vi "MGCC_StaEst_idx2pha.vi"(1 "n":dbl, 2 "Index":dbl[](array[numeric])) -> (0 "byphase":dbl[][](array[numeric]))   [LabVIEW 2016]
uses:
  <vilib>/imath/engines/lvmath2/RunTimeEngine/BitwiseOperatorToken/NIMS_Bitwise_Operator_And.vi
  <instcachedir>/0/NIMS_Bitwise_Operator_And_D587B28D2F2E4A5ABF81AE0392B9AD1B.lvgen/NIMS_Bitwise_Operator_And_D587B28D2F2E4A5ABF81AE0392B9AD1B_001.vi
  <vilib>/imath/engines/lvmath2/RunTimeEngine/BuiltInFunctions/findnz/NIMS_[1o]_findnz(GRowV).vi
  <instcachedir>/0/NIMS_[1o]_findnz(GRowV)_1AF74843B4874134ADE908C0A4A72F3C.lvgen/NIMS_[1o]_findnz(GRowV)_1AF74843B4874134ADE908C0A4A72F3C_000.vi
  <vilib>/imathl/engines/lvmath/Functions/Error Handling/Create Error.vi
  <vilib>/imath/engines/lvmath2/RunTimeEngine/BuiltInFunctions/size/NIMS_I32=size(GRow,I32).vi
  <instcachedir>/0/NIMS_I32=size(GRow,I32)_ECB8D6BA8B644FAD9EC9BDD2BFE864D8.lvgen/NIMS_I32=size(GRow,I32)_ECB8D6BA8B644FAD9EC9BDD2BFE864D8_000.vi
  <vilib>/imath/engines/lvmath2/RunTimeEngine/BuiltInFunctions/zeros/NIMS_M=zeros(I32,I32).vi
  <vilib>/imath/engines/lvmath2/RunTimeEngine/ErrorHandling/NIMS_Create Error From Enums.vi
  <vilib>/imath/engines/lvmath2/RunTimeEngine/IndexRead/NIMS V(V).vi
  <instcachedir>/0/NIMS V(V)_298D9CB7BFEB42B8BC8D9C3C28AE8C70.lvgen/NIMS V(V)_298D9CB7BFEB42B8BC8D9C3C28AE8C70_000.vi
  <vilib>/imath/engines/lvmath2/RunTimeEngine/IndexReplace/NIMS M(V,S)=V.vi
  <instcachedir>/0/NIMS M(V,S)=V_F75C9F1BFECF4A57AE59A9C096BE65FD.lvgen/NIMS M(V,S)=V_F75C9F1BFECF4A57AE59A9C096BE65FD_000.vi
  <vilib>/imath/engines/lvmath2/RunTimeEngine/IndexReplace/NIMS M(V,S)=S.vi
  <instcachedir>/0/NIMS M(V,S)=S_40CBAA0DA2C84D569C1A758010E9587E.lvgen/NIMS M(V,S)=S_40CBAA0DA2C84D569C1A758010E9587E_000.vi
  <vilib>/imath/engines/lvmath2/RunTimeEngine/NodeEndStatement/NIMS_NodeEndStatement_Output.vi
  <instcachedir>/0/NIMS_NodeEndStatement_Output_53EC0D466D134D7ABD903AC30B43404B.lvgen/NIMS_NodeEndStatement_Output_53EC0D466D134D7ABD903AC30B43404B_002.vi
  <vilib>/imath/engines/lvmath2/RunTimeEngine/ErrorHandling/NIMS_Finalize Error.vi
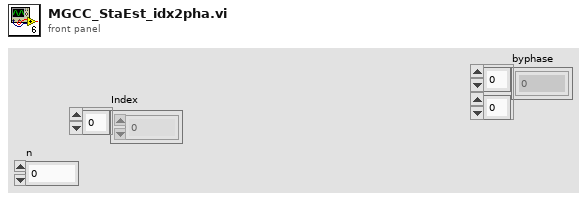
[diagram p1: front panel]
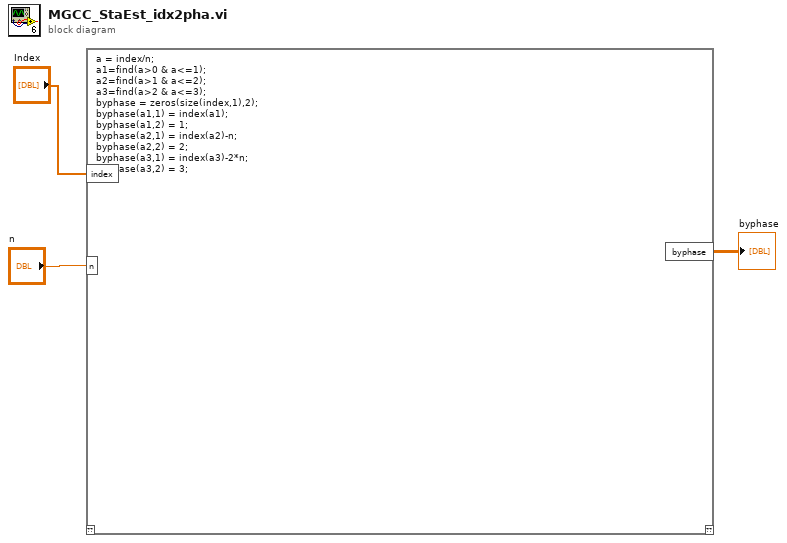
[diagram p0: block diagram]
diagram:
  n1 = mathscript code="a = index/n;\na1=find(a>0 & a<=1);\na2=find(a>1 & a<=2);\na3=find(a>2 & a<=3);\nbyphase = zeros(size(index,1),2);\nbyphase(a1,1) = index(a1);\nbyphase(a1,2) = 1;\nbyphase(a2,1) = index(a2)-n;\nbyphase(a2,2) = 2;\nbyphase(a3,1) = index(a3)-2*n;\nbyphase(a3,2) = 3;"("index"="Index", "n"="n") -> ("byphase"=→"byphase":dbl[][])  [unwired: 1 in, 1 out]
